vi "WBRT Controller Backup.vi"(6 "Spin up time":dbl, 7 "Manual Motor Control":bool, 8 "error in (no error)":errorcluster, 11 "WBRT State In":T2={"Encoders"={"Roll"=0.0, "Pitch"=0.0, "Yaw"=0.0, "Roll Trim"=0.0, "Pitch Trim"=0.0, "Yaw Trim"=0.0, "Roll Rate"=0.0, "Pitch Rate"=0.0, "Yaw Rate"=0.0}, "SPI Data"={"X-Gyro"=0.0, "Y-Gyro"=0.0, "Z-Gyro"=0.0, "X-Accel"=0.0, "Y-Accel"=0.0, "Z-Accel"=0.0}, "Camera"={"Numeric"=0.0}, "Filter Data"={"Filter Enabled?"=FALSE, "Filter Type"=enum."Equi-Ripple", "Pass Frequency"=1.0, "Stop Frequency (Equi-Ripple)"=0.45000000000000007, "Order"=0, "Ripple (dB)"=2.0}, "FPGA VI Reference"=refnum, "dt"=0.0, "Elapsed Time (msec)"=0, "Setpoints"={"Roll Setpoint"=125.0, "Pitch Setpoint"=125.0, "Yaw Setpoint"=125.0}, "Commands"={"Left Command"=0.0, "Right Command"=0.0}, "Trajectory Data"=[], "Gains"={"Gain1"=0.0, "Gain2"=0.0, "Gain3"=0.0, "Gain4"=0.0, "Gain5"=0.0, "Gain6"=0.0, "Gain7"=0.0, "Gain8"=0.0, "Gain9"=0.0}, "Global Variables"={"Variable1"=[], "Variable2"=[], "Variable3"=[], "Variable4"=[]}, "Centroid"={"X Centroid"=0.0, "Y Centroid"=0.0}, "Error1"=0.0, "Error2"=0.0, "Error3"=0.0, "Error4"=0.0, "Recorded Data"=[], "Landing Factor"=0.0} {"Trajectory Data" format="%0.3f"; "Filter Data"."Stop Frequency (Equi-Ripple)" format="%0.3f"; "Filter Data"."Pass Frequency" format="%0.3f"}) -> (0 "error out":errorcluster, 3 "WBRT State Out":T2={"Encoders"={"Roll"=0.0, "Pitch"=0.0, "Yaw"=0.0, "Roll Trim"=0.0, "Pitch Trim"=0.0, "Yaw Trim"=0.0, "Roll Rate"=0.0, "Pitch Rate"=0.0, "Yaw Rate"=0.0}, "SPI Data"={"X-Gyro"=0.0, "Y-Gyro"=0.0, "Z-Gyro"=0.0, "X-Accel"=0.0, "Y-Accel"=0.0, "Z-Accel"=0.0}, "Camera"={"Numeric"=0.0}, "Filter Data"={"Filter Enabled?"=FALSE, "Filter Type"=enum."Equi-Ripple", "Pass Frequency"=1.0, "Stop Frequency (Equi-Ripple)"=0.45000000000000007, "Order"=0, "Ripple (dB)"=2.0}, "FPGA VI Reference"=refnum, "dt"=0.0, "Elapsed Time (msec)"=0, "Setpoints"={"Roll Setpoint"=125.0, "Pitch Setpoint"=125.0, "Yaw Setpoint"=125.0}, "Commands"={"Left Command"=0.0, "Right Command"=0.0}, "Trajectory Data"=[], "Gains"={"Gain1"=0.0, "Gain2"=0.0, "Gain3"=0.0, "Gain4"=0.0, "Gain5"=0.0, "Gain6"=0.0, "Gain7"=0.0, "Gain8"=0.0, "Gain9"=0.0}, "Global Variables"={"Variable1"=[], "Variable2"=[], "Variable3"=[], "Variable4"=[]}, "Centroid"={"X Centroid"=0.0, "Y Centroid"=0.0}, "Error1"=0.0, "Error2"=0.0, "Error3"=0.0, "Error4"=0.0, "Recorded Data"=[], "Landing Factor"=0.0} {"Trajectory Data" format="%0.3f"; "Filter Data"."Stop Frequency (Equi-Ripple)" format="%0.3f"; "Filter Data"."Pass Frequency" format="%0.3f"}, 5 "Error Chart Data":T1)   [LabVIEW 2009]
doc: "This VI contains a mathscript node where a user must define a controller for the Whirlybird. All inputs are defined on the left edge of the mathscript node and the outputs are defined on the right. Users can still define other variables within the mathscript node.\n\nAuthor: Brandon Steele\n\nCopyright: Brigham Young University"
uses:
  Custom Controls/WBRT State.ctl
  Custom Controls/WBRT Encoders.ctl
  Custom Controls/WBRT SPI Data.ctl
  Custom Controls/WBRT Filter Data.ctl
  Custom Controls/WBRT Filter Type.ctl
  FPGA Samples/spi_single port_example/Host API/Controls/FPGA SPI_FPGA Ref.ctl
  Custom Controls/WBRT Setpoints.ctl
  Custom Controls/WBRT Commands.ctl
  Custom Controls/WBRT Gains.ctl
  Custom Controls/WBRT Global Variables.ctl
  <vilib>/imath/engines/lvmath2/RunTimeEngine/ErrorHandling/NIMS_Finalize Error.vi
  <vilib>/imath/engines/lvmath2/RunTimeEngine/Parser/MC_Version.vi
  <vilib>/imath/engines/lvmath2/RunTimeEngine/NodeEndStatement/NIMS_NodeEndStatement_Output.vi
  <instcachedir>/0/NIMS_NodeEndStatement_Output_B70DDD75627E4997AAE11E9955EDAA25.lvgen/NIMS_NodeEndStatement_Output_B70DDD75627E4997AAE11E9955EDAA25_000.vi
  <instcachedir>/0/NIMS_NodeEndStatement_Output_B70DDD75627E4997AAE11E9955EDAA25.lvgen/NIMS_NodeEndStatement_Output_B70DDD75627E4997AAE11E9955EDAA25_001.vi
  <vilib>/imath/engines/lvmath/Functions/Error Handling/MergeErrorsWrapper.vi
  <vilib>/imathl/engines/lvmath/Functions/Error Handling/Create Error.vi
  <vilib>/imath/engines/lvmath2/RunTimeEngine/BuiltInFunctions/eye/NIMS_M=eye(I32).vi
panel:
  # "Press Control + E to open block diagram\nor\nClick Window -> Show Block Diagram"
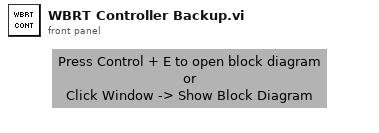
[diagram p1: front panel]
types:
  T1 = cluster{"[0]":dbl, "[1]":dbl, "[2]":dbl, "[3]":dbl, "[4]":dbl, "[5]":dbl, "[6]":dbl, "[7]":dbl, "[8]":dbl}
  T2 = typedef "WBRT State.ctl" = cluster{"Encoders":T3, "SPI Data":T4, "Camera":cluster{"Numeric":dbl}, "Filter Data":T5, "FPGA VI Reference":T7, "dt":dbl, "Elapsed Time (msec)":u32, "Setpoints":T8, "Commands":T9, "Trajectory Data":dbl[][], "Gains":T10, "Global Variables":T11, "Centroid":cluster{"X Centroid":sgl, "Y Centroid":sgl}, "Error1":dbl, "Error2":dbl, "Error3":dbl, "Error4":dbl, "Recorded Data":dbl[][], "Landing Factor":dbl}
  T3 = typedef "WBRT Encoders.ctl" = cluster{"Roll":dbl, "Pitch":dbl, "Yaw":dbl, "Roll Trim":dbl, "Pitch Trim":dbl, "Yaw Trim":dbl, "Roll Rate":dbl, "Pitch Rate":dbl, "Yaw Rate":dbl}
  T4 = typedef "WBRT SPI Data.ctl" = cluster{"X-Gyro":dbl, "Y-Gyro":dbl, "Z-Gyro":dbl, "X-Accel":dbl, "Y-Accel":dbl, "Z-Accel":dbl}
  T5 = typedef "WBRT Filter Data.ctl" = cluster{"Filter Enabled?":bool, "Filter Type":T6, "Pass Frequency":dbl, "Stop Frequency (Equi-Ripple)":dbl, "Order":i32, "Ripple (dB)":dbl}
  T6 = typedef "WBRT Filter Type.ctl" = enum16{"Equi-Ripple", "Butterworth", "Chebyshev"}
  T7 = typedef "FPGA SPI_FPGA Ref.ctl" = refnum<k20>
  T8 = typedef "WBRT Setpoints.ctl" = cluster{"Roll Setpoint":dbl, "Pitch Setpoint":dbl, "Yaw Setpoint":dbl}
  T9 = typedef "WBRT Commands.ctl" = cluster{"Left Command":dbl, "Right Command":dbl}
  T10 = typedef "WBRT Gains.ctl" = cluster{"Gain1":dbl, "Gain2":dbl, "Gain3":dbl, "Gain4":dbl, "Gain5":dbl, "Gain6":dbl, "Gain7":dbl, "Gain8":dbl, "Gain9":dbl}
  T11 = typedef "WBRT Global Variables.ctl" = cluster{"Variable1":dbl[][], "Variable2":dbl[][], "Variable3":dbl[][], "Variable4":dbl[][]}
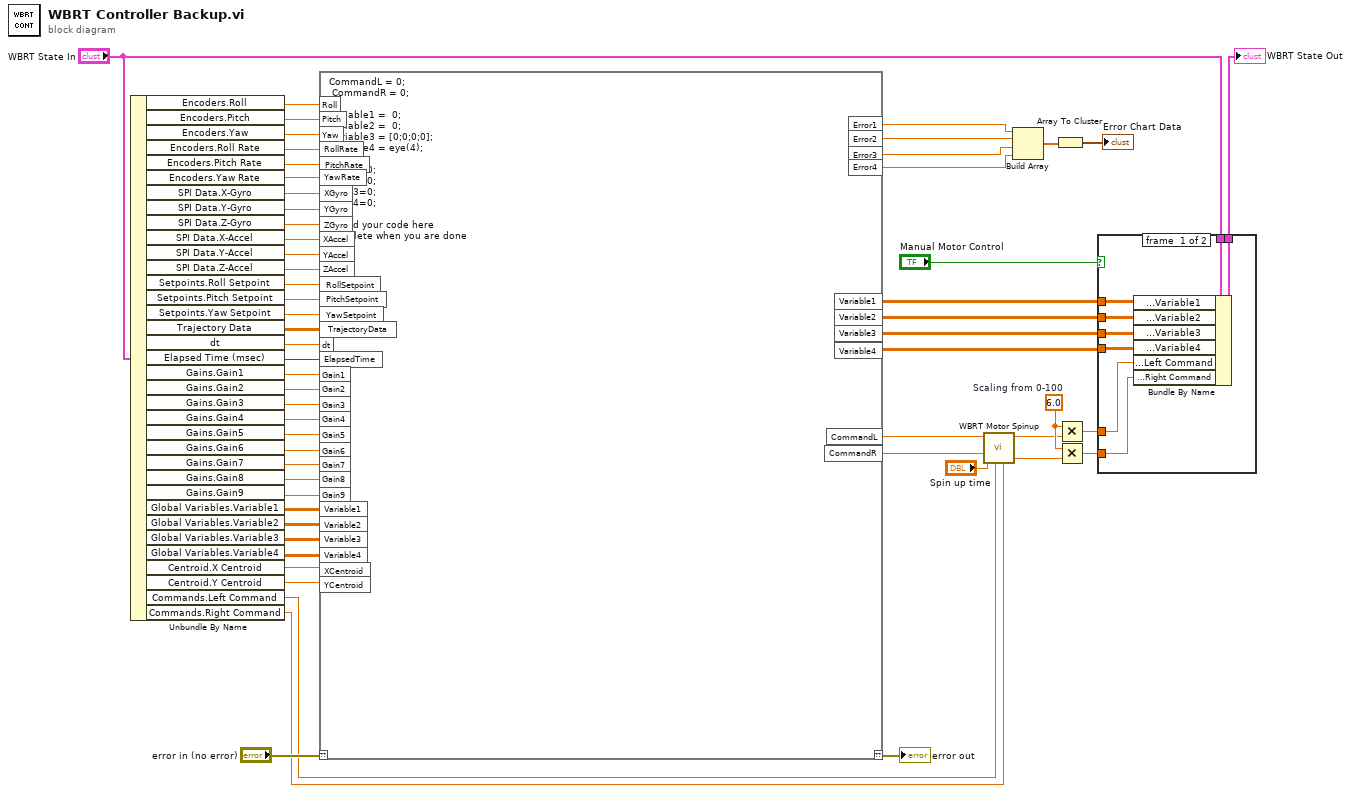
[diagram p0: block diagram]
diagram:
  w27 = 6.0  # Scaling from 0-100
  n1 = Unbundle By Name("WBRT State In") -> ("Encoders.Roll"=w58:dbl, "Encoders.Pitch"=w57:dbl, "Encoders.Yaw"=w56:dbl, "Encoders.Roll Rate"=w40:dbl, "Encoders.Pitch Rate"=w39:dbl, "Encoders.Yaw Rate"=w38:dbl, "SPI Data.X-Gyro"=w41:dbl, "SPI Data.Y-Gyro"=w55:dbl, "SPI Data.Z-Gyro"=w54:dbl, "SPI Data.X-Accel"=w53:dbl, "SPI Data.Y-Accel"=w52:dbl, "SPI Data.Z-Accel"=w51:dbl, "Setpoints.Roll Setpoint"=w46:dbl, "Setpoints.Pitch Setpoint"=w45:dbl, "Setpoints.Yaw Setpoint"=w44:dbl, "Trajectory Data"=w42:dbl[][], "dt"=w43:dbl, "Elapsed Time (msec)"=w2:u32, "Gains.Gain1"=w36:dbl, "Gains.Gain2"=w35:dbl, "Gains.Gain3"=w34:dbl, "Gains.Gain4"=w33:dbl, "Gains.Gain5"=w32:dbl, "Gains.Gain6"=w31:dbl, "Gains.Gain7"=w30:dbl, "Gains.Gain8"=w29:dbl, "Gains.Gain9"=w28:dbl, "Global Variables.Variable1"=w26:dbl[][], "Global Variables.Variable2"=w25:dbl[][], "Global Variables.Variable3"=w24:dbl[][], "Global Variables.Variable4"=w23:dbl[][], "Centroid.X Centroid"=w16:sgl, "Centroid.Y Centroid"=w15:sgl, "Commands.Left Command"=w10:dbl, "Commands.Right Command"=w9:dbl)
  n2 = mathscript code="CommandL = 0;\n CommandR = 0;\n \nVariable1 =  0;\nVariable2 =  0;\nVariable3 = [0;0;0;0];\nVariable4 = eye(4);\n\nError1=0;\nError2=0;\nError3=0;\nError4=0;\n\n% Add your code here\n% Delete when you are done\n\n%"("??"="error in (no error)", "Roll"=w58, "Pitch"=w57, "Yaw"=w56, "XGyro"=w41, "YGyro"=w55, "ZGyro"=w54, "XAccel"=w53, "YAccel"=w52, "ZAccel"=w51, "RollSetpoint"=w46, "PitchSetpoint"=w45, "YawSetpoint"=w44, "dt"=w43, "ElapsedTime"=w2, "TrajectoryData"=w42, "RollRate"=w40, "PitchRate"=w39, "YawRate"=w38, "Gain1"=w36, "Gain2"=w35, "Gain3"=w34, "Gain4"=w33, "Gain5"=w32, "Gain6"=w31, "Gain7"=w30, "Gain8"=w29, "Gain9"=w28, "Variable1"=w26, "Variable2"=w25, "Variable3"=w24, "Variable4"=w23, "XCentroid"=w16, "YCentroid"=w15) -> ("??"=→"error out":errorcluster, "CommandL"=w11:dbl, "CommandR"=w12:dbl, "Variable1"=w22:dbl[][], "Variable2"=w21:dbl[][], "Variable3"=w20:dbl[][], "Variable4"=w19:dbl[][], "Error1"=w8:dbl, "Error2"=w7:dbl, "Error3"=w6:dbl, "Error4"=w5:dbl)
  n3 = call "WBRT Motor Spinup.vi"("Previous loop Right Command"=w9, "Previous loop Left Command"=w10, "Spin up time"="Spin up time", "Current loop Right Command"=w12, "Current loop Left Command"=w11) -> ("Right Command"=w13:dbl, "Left Command"=w14:dbl)  [unwired: 5 in]
  n4 = Build Array(w8, w7, w6, w5) -> (w4:dbl[])
  n5 = Array To Cluster(array=w4) -> (cluster=→"Error Chart Data":T1)
  n6 = Multiply(x=w27, y=w14) -> (x*y=w18:dbl)
  n7 = Multiply(x=w27, y=w13) -> (x*y=w17:dbl)
  n8 = case shown="False" "Manual Motor Control" {
    tunnel: "WBRT State In" -> [w66 w67]
    tunnel: [w65 w67] -> w49
    tunnel: w22 -> [w64 _]
    tunnel: w21 -> [w63 _]
    tunnel: w20 -> [w62 _]
    tunnel: w19 -> [w61 _]
    tunnel: w18 -> [w59 _]
    tunnel: w17 -> [w60 _]
    frame #0 {
      n9 = Bundle By Name(cluster=w66, "Global Variables.Variable1"=w64, "Global Variables.Variable2"=w63, "Global Variables.Variable3"=w62, "Global Variables.Variable4"=w61, "Commands.Left Command"=w59, "Commands.Right Command"=w60) -> (w65:T2)
    }
    frame #1 {
    }
  }
  "WBRT State Out" <- w49
